vi "NMRvmefull2.vi"() -> ()   [LabVIEW 2013]
uses:
  <vilib>/Utility/file.llb/Read From Spreadsheet File (DBL).vi
  <vilib>/Analysis/NI_AALBase.lvlib
panel:
  out "Temperature":dbl(graph)=25.38
  out "+3V supply":dbl=3.026 format="%_4g"
  out "Temp (C)":dbl=25.38 format="%_4g"
  in  "RemovePed":bool=TRUE
  in  "IF / LOG Det":bool
  in  "Q curve file":string="realback213.txt"
  out "File name 2":string="C:\\users\\plm\\Desktop\\rssmt\\realback213.txt"
  in  "AutoBaseline":bool=TRUE
  out "RF OK":bool=TRUE
  out "Peak area (V-MHz)":sgl=0.009443471 format="%.3f"
  in  "Gauss Fit":bool=TRUE
  out "NMR Graph + Fit":cluster{cluster{dbl, "Numeric":dbl}[]}[](graph)=[{[{224.27, "Numeric"=0.0042339238095218485}, {224.274, "Numeric"=6.981333332070955e-05}, {224.27800000000002, "Numeric"=-0.0006870971428480408}, {224.282, "Numeric"=-0.0016368076190489793}, {224.286, "Numeric"=-0.00477931809524951}, {224.29000000000002, "Numeric"=0.005085371428580402}, {224.294, "Numeric"=-0.009742739047619882}, {224.298, "Numeric"=0.0019363504761802292}, {224.30200000000002, "Numeric"=-0.002977359999991209}, {224.306, "Numeric"=-0.005083870476190863}, {224.31, "Numeric"=-0.004883180952390091}, {224.31400000000002, "Numeric"=-0.005775291428562875}, {224.318, "Numeric"=0.0047397980952381055}, {224.322, "Numeric"=-0.006037912380960484}, {224.32600000000002, "Numeric"=0.0009915771428654077}, {224.33, "Numeric"=0.0006282666666670237}, {224.334, "Numeric"=0.00047215619046907443}, {224.33800000000002, "Numeric"=0.0001232457142936128}, {224.342, "Numeric"=-0.006618464761904125}, {224.346, "Numeric"=0.006747024761898569}, {224.35000000000002, "Numeric"=-0.003480285714278231}, {224.354, "Numeric"=0.0038996038095246606}, {224.358, "Numeric"=-0.002413306666672009}, {224.36200000000002, "Numeric"=-0.0019190171428501467}, {224.366, "Numeric"=-0.0005175276190466118}, {224.37, "Numeric"=-0.00020883809524264454}, {224.37400000000002, "Numeric"=0.008407051428577882}, {224.37800000000001, "Numeric"=0.000730140952382058}, {224.382, "Numeric"=0.01046043047618666}, {224.38600000000002, "Numeric"=0.008297920000005845}, {224.39000000000001, "Numeric"=0.009742609523810657}, {224.394, "Numeric"=0.017994499047615898}, {224.39800000000002, "Numeric"=0.0034535885714215495}, {224.40200000000002, "Numeric"=0.012919878095239203}, {224.406, "Numeric"=0.004093367619045088}, {224.41000000000003, "Numeric"=0.014774057142851372}, {224.41400000000002, "Numeric"=0.01516194666666768}, {224.418, "Numeric"=0.016157036190474202}, {224.42200000000003, "Numeric"=0.01785932571428113}, {224.42600000000002, "Numeric"=0.0043688152380961}, {224.43, "Numeric"=0.01998550476190326}, {224.43400000000003, "Numeric"=0.015509394285710826}, {224.43800000000002, "Numeric"=0.026640483809524457}, {224.442, "Numeric"=0.03537877333333226}, {224.44600000000003, "Numeric"=0.04492426285714046}, {224.45000000000002, "Numeric"=0.07197695238095274}, {224.454, "Numeric"=0.0846368419047612}, {224.45800000000003, "Numeric"=0.13880393142857003}, {224.46200000000002, "Numeric"=0.19827822095238096}, {224.466, "Numeric"=0.2987597104761901}, {224.47, "Numeric"=0.37234839999999964}, {224.47400000000002, "Numeric"=0.3509442895238092}, {224.478, "Numeric"=0.27274737904761887}, {224.482, "Numeric"=0.18105766857142902}, {224.48600000000002, "Numeric"=0.13467515809523728}, {224.49, "Numeric"=0.09199984761904763}, {224.494, "Numeric"=0.07433173714285841}, {224.49800000000002, "Numeric"=0.05667082666666532}, {224.502, "Numeric"=0.03731711619047632}, {224.506, "Numeric"=0.03617060571428774}, {224.51000000000002, "Numeric"=0.013731295238093306}, {224.514, "Numeric"=0.024399184761904936}, {224.518, "Numeric"=0.014474274285717006}, {224.52200000000002, "Numeric"=0.014656563809521234}, {224.526, "Numeric"=0.015646053333333507}, {224.53, "Numeric"=0.0029427428571462133}, {224.53400000000002, "Numeric"=0.019546632380949096}, {224.538, "Numeric"=0.005257721904762009}, {224.542, "Numeric"=0.011276011428575353}, {224.54600000000002, "Numeric"=0.005701500952376899}, {224.55, "Numeric"=0.007634190476190449}, {224.554, "Numeric"=0.0057740800000044305}, {224.55800000000002, "Numeric"=-0.0009788304761953592}, {224.562, "Numeric"=0.013975459047618832}, {224.566, "Numeric"=-0.0005630514285665486}, {224.57000000000002, "Numeric"=0.002105638095232318}, {224.574, "Numeric"=-0.0026184723809528523}, {224.578, "Numeric"=-0.002535382857137595}, {224.58200000000002, "Numeric"=0.007054906666659943}, {224.586, "Numeric"=-0.005447603809524597}, {224.59, "Numeric"=0.0092570857142913}, {224.59400000000002, "Numeric"=-0.006531024761912503}, {224.598, "Numeric"=-0.0043119352380963935}, {224.602, "Numeric"=-0.0028856457142798636}, {224.60600000000002, "Numeric"=-0.009752156190485008}, {224.61, "Numeric"=0.0027885333333317404}, {224.614, "Numeric"=-0.003763577142851095}, {224.61800000000002, "Numeric"=0.004191512380942419}, {224.622, "Numeric"=-0.009846198095240203}, {224.626, "Numeric"=0.0029232914285776145}, {224.63000000000002, "Numeric"=-0.0002000190476302063}, {224.63400000000001, "Numeric"=-0.0032161295238121905}, {224.638, "Numeric"=0.0013749600000062707}, {224.64200000000002, "Numeric"=-0.007126750476202895}, {224.64600000000002, "Numeric"=0.004378739047615762}, {224.65, "Numeric"=-0.005408571428565131}, {224.65400000000002, "Numeric"=0.0013113180952543488}, {224.65800000000002, "Numeric"=-0.0005615923809563516}, {224.662, "Numeric"=0.005572697142863395}, {224.66600000000003, "Numeric"=0.010414186666683532}, {224.67000000000002, "Numeric"=-0.0054371238095285235}]}, {[{224.27, "Numeric"=6.01501820042918e-80}, {224.274, "Numeric"=7.463635058397517e-77}, {224.27800000000002, "Numeric"=8.02951139199784e-74}, {224.282, "Numeric"=7.489504973441997e-71}, {224.286, "Numeric"=6.056788111780182e-68}, {224.29000000000002, "Numeric"=4.2467521990464116e-65}, {224.294, "Numeric"=2.581646246659611e-62}, {224.298, "Numeric"=1.3606982195033183e-59}, {224.30200000000002, "Numeric"=6.218020837729514e-57}, {224.306, "Numeric"=2.463586423195377e-54}, {224.31, "Numeric"=8.462695279325749e-52}, {224.31400000000002, "Numeric"=2.520431373319239e-49}, {224.318, "Numeric"=6.508281407086533e-47}, {224.322, "Numeric"=1.4570788056839866e-44}, {224.32600000000002, "Numeric"=2.8282971227566723e-42}, {224.33, "Numeric"=4.759839345816419e-40}, {224.334, "Numeric"=6.945201173055507e-38}, {224.33800000000002, "Numeric"=8.786231412260955e-36}, {224.342, "Numeric"=9.637085620884255e-34}, {224.346, "Numeric"=9.164611719697454e-32}, {224.35000000000002, "Numeric"=7.556273944588158e-30}, {224.354, "Numeric"=5.401651874678868e-28}, {224.358, "Numeric"=3.34788676622809e-26}, {224.36200000000002, "Numeric"=1.799037442911426e-24}, {224.366, "Numeric"=8.38175411368294e-23}, {224.37, "Numeric"=3.385750120268754e-21}, {224.37400000000002, "Numeric"=1.1857691883269137e-19}, {224.37800000000001, "Numeric"=3.600565303913174e-18}, {224.382, "Numeric"=9.479086698960475e-17}, {224.38600000000002, "Numeric"=2.1636528004037594e-15}, {224.39000000000001, "Numeric"=4.2818743518635706e-14}, {224.394, "Numeric"=7.346923866671516e-13}, {224.39800000000002, "Numeric"=1.0929553797536967e-11}, {224.40200000000002, "Numeric"=1.409693174908673e-10}, {224.406, "Numeric"=1.576420356833665e-09}, {224.41000000000003, "Numeric"=1.5284271516595578e-08}, {224.41400000000002, "Numeric"=1.2848212948986133e-07}, {224.418, "Numeric"=9.364098652394221e-07}, {224.42200000000003, "Numeric"=5.917176272529978e-06}, {224.42600000000002, "Numeric"=3.24181558725535e-05}, {224.43, "Numeric"=0.0001539881769482936}, {224.43400000000003, "Numeric"=0.0006341788018151727}, {224.43800000000002, "Numeric"=0.00226444270765884}, {224.442, "Numeric"=0.007010293895939192}, {224.44600000000003, "Numeric"=0.018816393476206752}, {224.45000000000002, "Numeric"=0.043788676523356475}, {224.454, "Numeric"=0.08835121465093783}, {224.45800000000003, "Numeric"=0.15455693697092934}, {224.46200000000002, "Numeric"=0.23441735009928816}, {224.466, "Numeric"=0.30825936159556316}, {224.47, "Numeric"=0.351453659177543}, {224.47400000000002, "Numeric"=0.34741225678765525}, {224.478, "Numeric"=0.2977470558073471}, {224.482, "Numeric"=0.221245826707288}, {224.48600000000002, "Numeric"=0.14253711737890468}, {224.49, "Numeric"=0.07961705843383239}, {224.494, "Numeric"=0.038557561204089354}, {224.49800000000002, "Numeric"=0.01618967973809184}, {224.502, "Numeric"=0.005893757070405926}, {224.506, "Numeric"=0.0018602507007593632}, {224.51000000000002, "Numeric"=0.0005090682305821025}, {224.514, "Numeric"=0.0001207829924597174}, {224.518, "Numeric"=2.4846249844449873e-05}, {224.52200000000002, "Numeric"=4.431402343942447e-06}, {224.526, "Numeric"=6.85246443976148e-07}, {224.53, "Numeric"=9.187083639661259e-08}, {224.53400000000002, "Numeric"=1.0679079566260783e-08}, {224.538, "Numeric"=1.0762551601872471e-09}, {224.542, "Numeric"=9.404201878403823e-11}, {224.54600000000002, "Numeric"=7.124492154518162e-12}, {224.55, "Numeric"=4.679626094170481e-13}, {224.554, "Numeric"=2.6649782428300915e-14}, {224.55800000000002, "Numeric"=1.3158350599636148e-15}, {224.562, "Numeric"=5.63293204866455e-17}, {224.566, "Numeric"=2.090705410024211e-18}, {224.57000000000002, "Numeric"=6.727852261849235e-20}, {224.574, "Numeric"=1.8770909748198122e-21}, {224.578, "Numeric"=4.5406650789039826e-23}, {224.58200000000002, "Numeric"=9.523111943662686e-25}, {224.586, "Numeric"=1.7316638147306155e-26}, {224.59, "Numeric"=2.73006851679074e-28}, {224.59400000000002, "Numeric"=3.731717711700825e-30}, {224.598, "Numeric"=4.42251478291779e-32}, {224.602, "Numeric"=4.544175282554456e-34}, {224.60600000000002, "Numeric"=4.0482388575633574e-36}, {224.61, "Numeric"=3.1268169365028866e-38}, {224.614, "Numeric"=2.0939391382554106e-40}, {224.61800000000002, "Numeric"=1.2157686085224232e-42}, {224.622, "Numeric"=6.120164128543997e-45}, {224.626, "Numeric"=2.671163581143564e-47}, {224.63000000000002, "Numeric"=1.0107952049122365e-49}, {224.63400000000001, "Numeric"=3.316279555131142e-52}, {224.638, "Numeric"=9.433315641894263e-55}, {224.64200000000002, "Numeric"=2.3264990067670043e-57}, {224.64600000000002, "Numeric"=4.9746971738274e-60}, {224.65, "Numeric"=9.222649391143447e-63}, {224.65400000000002, "Numeric"=1.4824157514032807e-65}, {224.65800000000002, "Numeric"=2.0659015212002933e-68}, {224.662, "Numeric"=2.496171856005559e-71}, {224.66600000000003, "Numeric"=2.6149574193251713e-74}, {224.67000000000002, "Numeric"=2.375089791147989e-77}]}]
  in  "Amp of Q curve":dbl=2.899999999999994 min=0.0 max=3.0 step=0.01 format="%_3f"
  in  "Subtract Q curve":bool=TRUE
  in  "Adjust Tune":bool
  out "Ped Offset":dbl(graph)=-0.035859999999999656
  out "Pedestal Difference":dbl(graph)=0.0002877333333277249
  out "# Good Spectra":i32=99
  in  "Quality cuts":bool=TRUE
  out "Pedestal OK":bool=TRUE
  out "Sweep #":i32=40
  out "1st Sweep":bool
  out "ADC volts OK":bool=TRUE
  out "Peak Height Distribution":cluster{"Y":dbl[], "Y":dbl[]}[](graph)=[{"Y"=[0.33833505051969587, 0.33850925906127166, 0.33868346760284745, 0.33885767614442325, 0.3390318846859991, 0.3392060932275749, 0.3393803017691507, 0.3395545103107265, 0.33972871885230227, 0.33990292739387806, 0.34007713593545386, 0.3402513444770297, 0.3404255530186055, 0.3405997615601813, 0.3407739701017571, 0.3409481786433329, 0.34112238718490867, 0.34129659572648446, 0.3414708042680603, 0.3416450128096361, 0.3418192213512119, 0.3419934298927877, 0.3421676384343635, 0.3423418469759393, 0.3425160555175151, 0.3426902640590909, 0.3428644726006667, 0.3430386811422425, 0.3432128896838183, 0.3433870982253941, 0.3435613067669699, 0.3437355153085457, 0.34390972385012153, 0.3440839323916973, 0.3442581409332731, 0.3444323494748489, 0.3446065580164247, 0.3447807665580005, 0.3449549750995763, 0.34512918364115214, 0.34530339218272793, 0.3454776007243037, 0.3456518092658795, 0.3458260178074553, 0.3460002263490311, 0.3461744348906069, 0.34634864343218275, 0.34652285197375854, 0.34669706051533433, 0.3468712690569101, 0.3470454775984859, 0.3472196861400617, 0.3473938946816375, 0.3475681032232133, 0.34774231176478915, 0.34791652030636494, 0.34809072884794073, 0.3482649373895165, 0.3484391459310923, 0.3486133544726681, 0.3487875630142439, 0.34896177155581976, 0.34913598009739555, 0.34931018863897134, 0.34948439718054713, 0.34965860572212293, 0.3498328142636987, 0.3500070228052745, 0.35018123134685036, 0.35035543988842616, 0.35052964843000195, 0.35070385697157774, 0.35087806551315354, 0.35105227405472933, 0.3512264825963051, 0.35140069113788097, 0.35157489967945676, 0.35174910822103256, 0.35192331676260835, 0.35209752530418414, 0.35227173384575994, 0.35244594238733573, 0.3526201509289116, 0.3527943594704874, 0.35296856801206317, 0.35314277655363896, 0.35331698509521475, 0.35349119363679055, 0.35366540217836634, 0.3538396107199422, 0.354013819261518, 0.3541880278030938, 0.35436223634466957, 0.35453644488624536, 0.35471065342782115, 0.35488486196939695, 0.3550590705109728, 0.3552332790525486, 0.3554074875941244, 0.3555816961357002], "Y"=[1.0, 0.0, 0.0, 0.0, 0.0, 0.0, 0.0, 0.0, 0.0, 0.0, 1.0, 0.0, 0.0, 0.0, 0.0, 0.0, 0.0, 0.0, 0.0, 0.0, 2.0, 0.0, 0.0, 0.0, 1.0, 0.0, 0.0, 1.0, 0.0, 1.0, 0.0, 1.0, 3.0, 0.0, 0.0, 3.0, 1.0, 2.0, 3.0, 3.0, 1.0, 1.0, 3.0, 4.0, 3.0, 2.0, 4.0, 0.0, 3.0, 0.0, 2.0, 1.0, 3.0, 0.0, 4.0, 2.0, 4.0, 0.0, 4.0, 2.0, 1.0, 0.0, 0.0, 1.0, 1.0, 2.0, 1.0, 1.0, 2.0, 0.0, 2.0, 1.0, 4.0, 1.0, 0.0, 1.0, 2.0, 2.0, 0.0, 0.0, 3.0, 0.0, 0.0, 1.0, 1.0, 0.0, 0.0, 0.0, 1.0, 0.0, 0.0, 0.0, 0.0, 0.0, 0.0, 0.0, 1.0, 1.0, 2.0, 1.0]}]
  in  "# of Sweeps":i32=1000
  out "Std Dev (V)":dbl=0.003420750735864373 format="%_2g"
  out "Peak mean (V)":dbl=0.3477737466927863 format="%_4g"
  out "Peak Height":dbl(graph)=0.3558827955311164
  in  "Raw Data":bool=TRUE
  in  "Tank RF":bool=TRUE
  in  "IF Atten (dB)":i8 min=0 max=31 step=1
  in  "IFoffset (V)":dbl=-1.2985525999999998 min=-5.0 max=5.0 step=0.001 format="%.4f"
  in  "Tune  (V)":dbl=1.091700000000001 min=0.0 max=5.0 step=0.001 format="%.4f"
  in  "Hi / Lo IF Gain":bool
  out "Voltage Array":sgl[](array[numeric])=[0.0865, 0.0777, 0.0724, 0.067, 0.0595, 0.0651, 0.0461, 0.0537, 0.0448, 0.0388, 0.0352, 0.0306, 0.0375, 0.0232, 0.0268, 0.0231, 0.0197, 0.0162, 0.0064, 0.0168, 0.0037, 0.0083, -0.0007, -0.0028, -0.0039, -0.006, 0.0003, -0.0096, -0.002, -0.0062, -0.0067, -0.0003, -0.0166, -0.0088, -0.0192, -0.01, -0.011, -0.0113, -0.0108, -0.0254, -0.0108, -0.0162, -0.0059, 0.0021, 0.011, 0.0375, 0.0497, 0.1035, 0.1627, 0.263, 0.3365, 0.3151, 0.237, 0.1455, 0.0994, 0.0571, 0.0399, 0.0228, 0.0041, 0.0037, -0.0179, -0.0063, -0.0152, -0.0139, -0.0117, -0.0231, -0.0051, -0.0179, -0.0103, -0.0142, -0.0105, -0.0105, -0.0153, 0.0017, -0.0107, -0.0058, -0.0082, -0.0057, 0.0064, -0.0035, 0.0139, 0.0009, 0.006, 0.0104, 0.0066, 0.0223, 0.019, 0.0303, 0.0197, 0.036, 0.0365, 0.0372, 0.0456, 0.041, 0.0565, 0.0508, 0.0617, 0.0641, 0.0746, 0.0839, 0.0726] format="%.4f"
  in  "Invert Polarity":bool
  out "Pedestal Diff (V)":sgl=0.00028773333 format="%.3f"
  out "Peak amp (V)":sgl=0.3558828 format="%.3f"
  in  "Save Data to File":bool
  in  "RF Level (dBm)":dbl=-1.0 min=-10.0 max=1.0 step=0.1 format="%.2f"
  out "SMT error out":errorcluster
  out "Sample RMS (V)":dbl=0.01090891089108911 format="%.4f"
  in  "# Sample/step":i32=100 min=1 max=1000 step=100
  in  "Step Width (MHz)":dbl=0.004 min=0.0 max=1000.0 step=0.0005 format="%.4f"
  in  "Freq Span (MHz)":dbl=0.4 min=0.0 max=3000.0 step=0.1 format="%.3f"
  in  "Center Freq (MHz)":dbl=224.47 min=0.005 max=6000.0 step=0.1 format="%.3f"
  in  "Sweep Mode":u16(ring)=3 items=["Off", "Single", "Auto", "Step"]
  in  "GPIB Addr (28)":refnum<visa-resource-name>="GPIB0::28::INSTR"
  # "Settings"
  # "E1039 Prototype NMR Control Panel"
  # "D\nA\nC"
  # "R\nF\n\nG\nE\nN \n\n+\n\nI\nF"
  # "A\nD\nC"
  # "D\nA\nT\nA"
  # "I\n/\nO"
  # "Results"
  # "A\nv\ne\nr\na\ng\ne"
  # "S\nw\ne\ne\np"
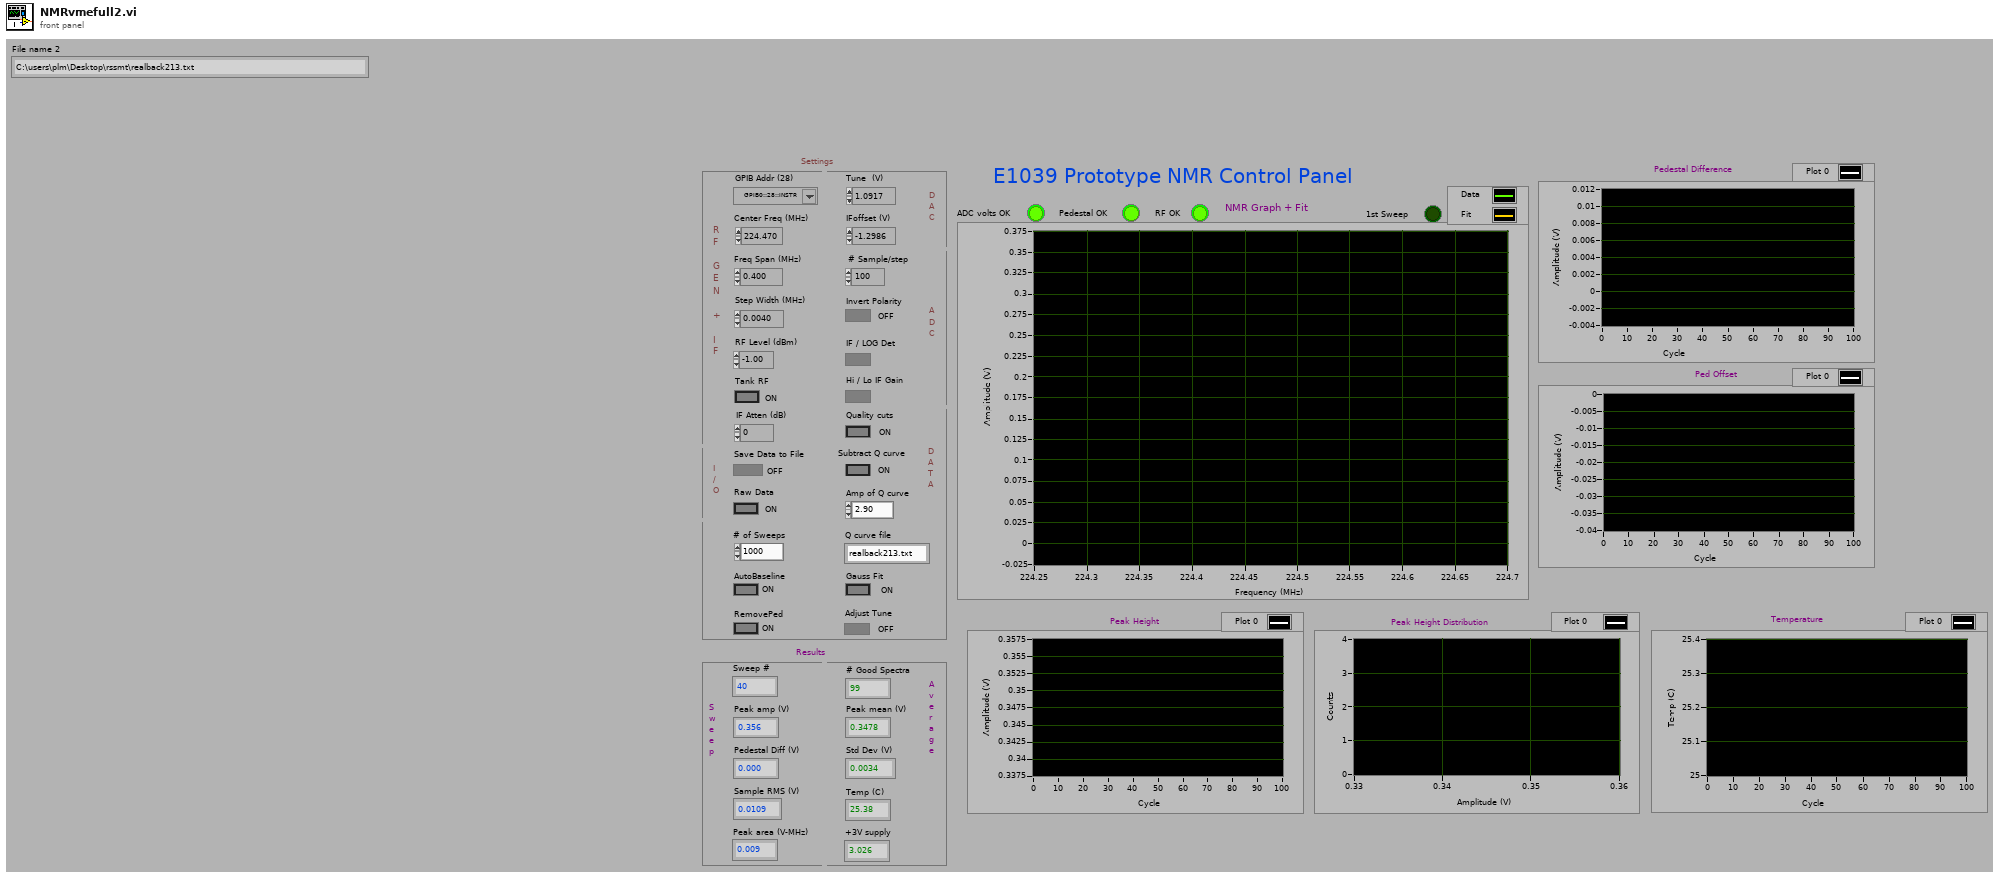
[diagram p1: front panel]
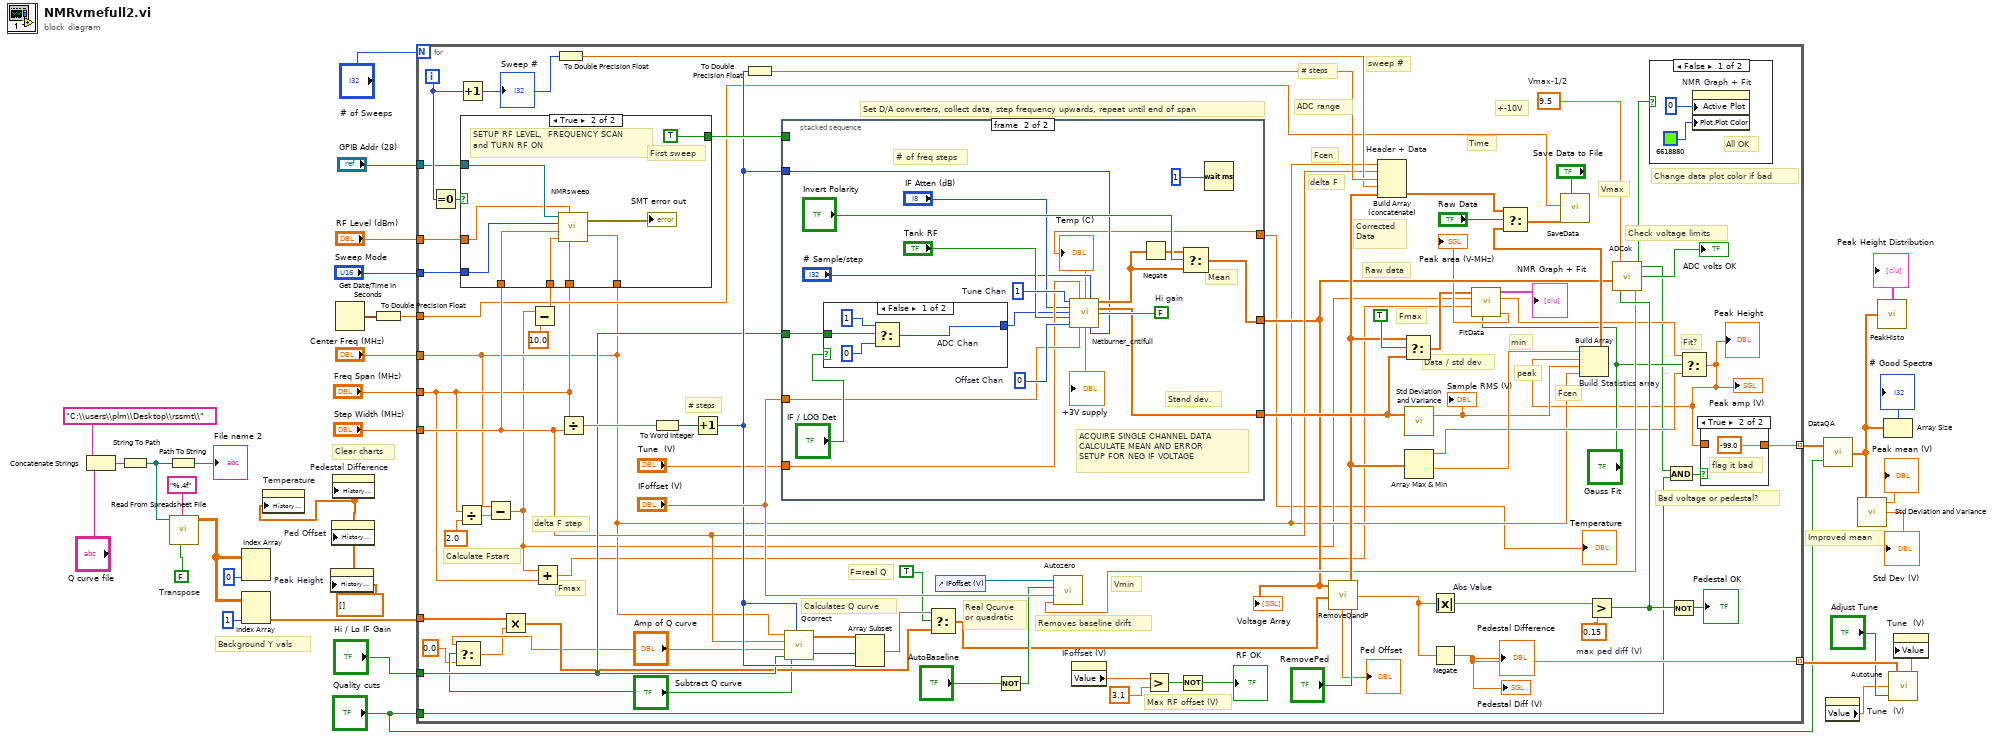
[diagram p0: block diagram]
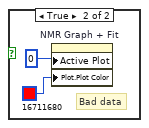
[diagram p2: hidden frame]
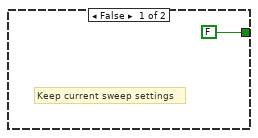
[diagram p4: hidden frame]
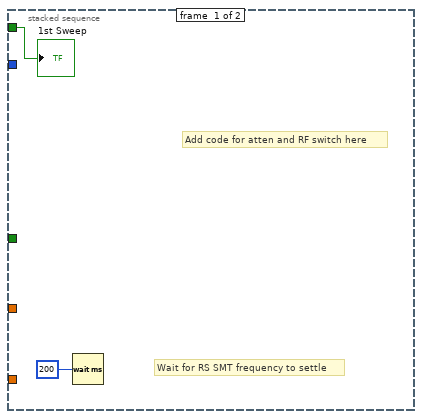
[diagram p5: hidden frame]
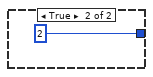
[diagram p6: hidden frame]
diagram:
  w9 = FALSE  # Transpose
  w1 = dbl[] []
  # "Background Y vals"
  # "Clear charts"
  # "Improved mean"
  n1 = Concatenate Strings "Concatenate Strings"("C:\\users\\plm\\Desktop\\rssmt\\", "Q curve file") -> (w12:string)
  n2 = String To Path(string=w12) -> (path=w8:path)
  n3 = Path To String(path=w8) -> (string=→"File name 2":string)
  n4 = call-poly <vilib>:"Read From Spreadsheet File.vi"("transpose (no:F)"=w9, "format (%.3f)"="%.4f", "file path (dialog if empty)"=w8) -> ("all rows"=w7:dbl[][])  [unwired: 4 in, 4 out]
  n5 = Index Array "Index Array"(array=w7, index (col)=0) -> ()  [unwired: 1 in, 1 out]
  n6 = Index Array(array=w7, index (col)=1) -> (element=w2:dbl[])  [unwired: 1 in]
  n7 = property on="Temperature" class="WFChart (strict)"("History Data"=w1) -> ()  [unwired: 2 in, 2 out]
  n8 = property on="Peak Height" class="WFChart (strict)"("History Data"=w1) -> ()  [unwired: 2 in, 2 out]
  n9 = property on="Ped Offset" class="WFChart (strict)"("History Data"=w1) -> ()  [unwired: 2 in, 2 out]
  n10 = property on="Pedestal Difference" class="WFChart (strict)"("History Data"=w1) -> ()  [unwired: 2 in, 2 out]
  n11 = Get Date/Time In Seconds() -> (seconds since 1Jan1904=w14:timestamp)
  n12 = To Double Precision Float(number=w14) -> (double precision float=w13:dbl)
  n13 = for {
    N: "# of Sweeps" -> [_]
    tunnel: [w94] -> w29 mode=indexing
    tunnel: "Quality cuts" -> [w71]
    tunnel: [w77] -> w26 mode=indexing
    tunnel: "Center Freq (MHz)" -> [w58]
    tunnel: "Freq Span (MHz)" -> [w64]
    tunnel: "Step Width (MHz)" -> [w70]
    tunnel: "Sweep Mode" -> [w81]
    tunnel: "Hi / Lo IF Gain" -> [w80]
    tunnel: "GPIB Addr (28)" -> [w79]
    tunnel: "RF Level (dBm)" -> [w78]
    tunnel: w13 -> [w65]
    tunnel: w2 -> [w43]
    i -> [w92]
    w75 = 9.5  # Vmax-1/2
    w95 = 0.15  # max ped diff (V)
    # "F=real Q"
    # "Real Qcurve\nor quadratic"
    # "+-10V"
    # "Vmax"
    # "Change data plot color if bad"
    # "Max RF offset (V)"
    # "Fmax"
    # "Fit?"
    # "Fmax"
    # "Time"
    # "Vmin"
    # "min"
    # "peak"
    # "Raw data"
    # "Corrected\nData"
    # "Fcen"
    # "delta F"
    # "# steps"
    # "ADC range"
    # "sweep #"
    # "Fcen"
    # "Set D/A converters, collect data, step frequency upwards, repeat until end of span"
    # "Calculates Q curve"
    # "Removes baseline drift"
    # "Bad voltage or pedestal?"
    # "Check voltage limits"
    # "Data / std dev"
    # "# steps"
    # "Calculate Fstart"
    # "delta F step"
    n14 = Equal To 0?(x=w92) -> (x = 0?=w97:bool)
    n15 = Select(t="Amp of Q curve", s="Subtract Q curve", f=0.0) -> (s? t:f=w38:dbl)
    n16 = Divide(x=w64, y=sgl 2.0) -> (x/y=w108:dbl)
    n17 = Increment(x=w92) -> (x+1=w82:i32)
    "Sweep #" <- w82
    n18 = Subtract(x=w58, y=w108) -> (x-y=w53:dbl)
    n19 = Multiply(x=w43, y=w38) -> (x*y=w42:dbl[])
    n20 = Subtract(x=w53, y=10.0) -> (x-y=w106:dbl)
    n21 = case shown="True" w97 {
      tunnel: w106 -> [_ w126]
      tunnel: w70 -> [_ w124]
      tunnel: w58 -> [_ w123]
      tunnel: w64 -> [_ w125]
      tunnel: [FALSE TRUE] -> w96
      tunnel: w81 -> [_ w120]
      tunnel: w79 -> [_ w119]
      tunnel: w78 -> [_ w118]
      frame False {
        # "Keep current sweep settings"
      }
      frame True {
        # "First sweep"
        # "SETUP RF LEVEL,  FREQUENCY SCAN\nand TURN RF ON"
        n22 = call "NMRsweep.vi"("Center Freq (MHz)"=w123, "Freq Span (MHz)"=w125, "RF Level (dBm)"=w118, "Foffset (MHz)"=w126, "Step Width (MHz)"=w124, "Sweep Mode"=w120, "GPIB Addr (28)"=w119) -> ("error out"=→"SMT error out":errorcluster)
      }
    }
    n23 = Add(x=w53, y=w64) -> (x+y=w52:dbl)
    n24 = To Double Precision Float(number=w82) -> (double precision float=w83:dbl)
    n25 = Divide(x=w64, y=w70) -> (x/y=w110:dbl)
    n26 = To Word Integer(number=w110) -> (16bit integer=w107:i16)
    n27 = Increment(x=w107) -> (x+1=w86:i16)
    n28 = To Double Precision Float(number=w86) -> (double precision float=w85:dbl)
    n29 = stacked-sequence {
      tunnel: [_ w134] -> w100
      tunnel: [_ w146] -> w68
      tunnel: w86 -> [_ w131]
      tunnel: "IFoffset (V)" -> [_ w141]
      tunnel: w80 -> [_ w144]
      tunnel: w96 -> [w127 _]
      tunnel: "Tune  (V)" -> [_ w139]
      tunnel: [_ w129] -> w34
      frame #0 {
        # "Add code for atten and RF switch here"
        # "Wait for RS SMT frequency to settle"
        n30 = Wait (ms)(milliseconds to wait=200) -> ()  [unwired: 1 out]
        "1st Sweep" <- w127
      }
      frame #1 {
        w136 = FALSE  # Hi gain
        w142 = 0  # Offset Chan
        w140 = 1  # Tune Chan
        # "Stand dev."
        # "Mean"
        # "ACQUIRE SINGLE CHANNEL DATA\nCALCULATE MEAN AND ERROR\nSETUP FOR NEG IF VOLTAGE"
        # "# of freq steps"
        n31 = case shown="False" "IF / LOG Det" {
          tunnel: w144 -> [w152 _]
          tunnel: [w149 2] -> w133
          frame False {
            n32 = Select "ADC Chan"(t=1, s=w152, f=0) -> (s? t:f=w149:i32)
          }
          frame True {
          }
        }
        n33 = call "Netburner_cntlfull.vi"("Tune DAC"=w140, "Tune Volt"=w139, "# Data"="# Sample/step", "IF Atten (dB)"="IF Atten (dB)", "NMR ADC"=w133, "Hi Gain"=w136, "Tank RF"="Tank RF", "Offset DAC"=w142, "Offset Volt"=w141, "# f steps"=w131) -> ("Temp (C)"=w129:dbl, "ADC value"=w135:dbl[], "ADC error"=w134:dbl[], "Volts"=→"+3V supply":dbl)  [unwired: 2 out]
        "Temp (C)" <- w129
        n34 = Negate(x=w135) -> (-x=w145:dbl[])
        n35 = Select(t=w145, s="Invert Polarity", f=w135) -> (s? t:f=w146:dbl[])
        n36 = Wait (ms)(milliseconds to wait=1) -> ()  [unwired: 1 out]
      }
    }
    "Voltage Array" <- w68
    "Temperature" <- w34
    n37 = call "Qcorrect.vi"("Subtract Q curve"="Subtract Q curve", "Nstep"=w86, "IF or Log"=w80, "Amp of Q curve"="Amp of Q curve", "Step Width (MHz)"=w70, "Center Freq (MHz)"=w58) -> ("Start"=w101:i32, "Array"=w102:dbl[])
    n38 = Array Subset "Array Subset"(array=w102, index=w101, length=w86) -> (w46:dbl[])
    n39 = Select(t=w46, s=TRUE, f=w42) -> (s? t:f=w45:dbl[])
    n40 = control-ref of="IFoffset (V)"() -> (w74:refnum<vi>)
    n41 = Not(x="AutoBaseline") -> (.not. x?=w47:bool)
    n42 = property on="IFoffset (V)" class="DigNum (strict)"() -> ("Value"=w62:dbl)  [unwired: 2 in, 2 out]
    n43 = Greater?(x=w62, y=3.1) -> (0:w60:bool)
    n44 = Not(x=w60) -> (.not. x?=→"RF OK":bool)
    n45 = call "RemoveQandP.vi"("Subtract Ped?"="RemovePed", "Qcurve"=w45, "Raw data"=w68) -> ("Ped L-R"=w88:dbl, "Corrected data"=w84:dbl[], "Ped Offfset"=→"Ped Offset":dbl)
    n46 = Build Array (concatenate) "Header + Data"(w58, w70, w85, w83, w84) -> (w87:dbl[])
    n47 = Select(t=w84, s=TRUE, f=w100) -> (s? t:f=w54:dbl[])
    n48 = call <vilib>:"Std Deviation and Variance.vi"("X"=w100) -> ("mean"=w69:dbl)  [unwired: 1 in, 2 out]
    "Sample RMS (V)" <- w69
    n49 = Array Max & Min(array=w84) -> (max value=w63:dbl, min value=w99:dbl)  [unwired: 2 out]
    n50 = Absolute Value "Abs Value"(x=w88) -> (abs(x)=w90:dbl)
    n51 = Negate(x=w88) -> (-x=w77:dbl)
    "Pedestal Diff (V)" <- w77
    "Pedestal Difference" <- w77
    n52 = call "FitData.vi"("Fit?"="Gauss Fit", "Fmax"=w52, "Fmin"=w53, "Yarray"=w54) -> ("Peak Area (V-MHz)"=→"Peak area (V-MHz)":dbl, "Amplitude (V)"=w56:dbl, "NMR Graph + Fit"=→"NMR Graph + Fit":cluster{cluster{dbl, "Numeric":dbl}[]}[])  [unwired: 2 out]
    n53 = Greater?(x=w90, y=w95) -> (0:w76:bool)
    n54 = call "ADCok.vi"("PedOK"=w76, "Array"=w68, "Vmax-1/2"=w75) -> ("Vmin"=w73:dbl, "ADC voltages OK"=→"ADC volts OK":bool, "Allok"=w50:bool)
    n55 = call "Autozero.vi"("Vmin (V)"=w73, "IFoffset (V)"="IFoffset (V)", "IF or Log"=w47, "reference"=w74) -> ()
    n56 = case shown="False" w50 {
      frame False {
        # "All OK"
        n57 = property on="NMR Graph + Fit" class="XYGraph (strict)"("Active Plot"=0, "Plot.Plot Color"=u32 6618880) -> ()  [unwired: 2 in, 2 out]
      }
      frame True {
        # "Bad data"
        n58 = property on="NMR Graph + Fit" class="XYGraph (strict)"("Active Plot"=0, "Plot.Plot Color"=u32 16711680) -> ()  [unwired: 2 in, 2 out]
      }
    }
    n59 = And(x=w50, y=w71) -> (x .and. y?=w91:bool)
    n60 = Not(x=w76) -> (.not. x?=→"Pedestal OK":bool)
    n61 = Select(t=w56, s="Gauss Fit", f=w63) -> (s? t:f=w49:dbl)
    "Peak amp (V)" <- w49
    "Peak Height" <- w49
    n62 = Build Array "Build Statistics array"(w99, w49, w69, w58) -> (w105:dbl[])
    n63 = Select(t=w87, s="Raw Data", f=w105) -> (s? t:f=w66:dbl[])
    n64 = call "SaveData.vi"("Array"=w66, "Save Data to File"="Save Data to File", "Ext time (sec)"=w65) -> ()  [unwired: 1 out]
    n65 = case shown="True" w91 {
      tunnel: [w115 -99.0] -> w94
      tunnel: w49 -> [w115 _]
      frame False {
        # "Data OK"
      }
      frame True {
        # "flag it bad"
      }
    }
  }
  n66 = call "DataQA.vi"("Quality cuts"="Quality cuts", "Data In"=w29) -> ("Data Out"=w28:dbl[])
  n67 = property on="Tune  (V)" class="DigNum (strict)"() -> ("Value"=w17:dbl)  [unwired: 2 in, 2 out]
  n68 = call <vilib>:"Std Deviation and Variance.vi"("X"=w28) -> ("mean"=→"Peak mean (V)":dbl, "standard deviation"=→"Std Dev (V)":dbl)  [unwired: 1 in, 1 out]
  n69 = call "PeakHisto.vi"("Data Out"=w28) -> ("XY Graph"=→"Peak Height Distribution":cluster{"Y":dbl[], "Y":dbl[]}[])
  n70 = Array Size(array=w28) -> (size(s)=→"# Good Spectra":i32)
  n71 = call "Autotune.vi"("Adjust Tune"="Adjust Tune", "Tune Vin"=w17, "Pedestal Diff"=w26) -> ("Tune Vout"=w16:dbl)
  n72 = property on="Tune  (V)" class="DigNum (strict)"("Value"=w16) -> ()  [unwired: 2 in, 2 out]
